vi "Host Main.vi"() -> ()   [LabVIEW 2014]
uses:
  rotate right.ctl
  rotate left.ctl
panel:
  in  "Rleft":T1
  in  "RRight":T2
  in  "Cancel Button":bool
  in  "Target IP Address":string="172.16.0.1"
  in  "Left Button":bool
  in  "Down Button":bool
  in  "Up Button":bool
  in  "Right Button":bool
  in  "Stop Button":bool
  # "Rover Demo (Host)"
  # "1. Confirm the IP address listed matches the WiFi IP address of the myRIO you are working with. Your myRIO has\ntwo different IP addresses, one for when it is connected through USB and another when it is broadcasting its own \nWiFi network.\n2. Open and Run the RT Main VI\n3. Run this VI\n4. Press all of the buttons and confirm they perform the appripriate movements."
  # "For help on troubleshooting this example as well as a brief description of how this example works \nvisit the help document under the My Computer section of the Project Viewer"
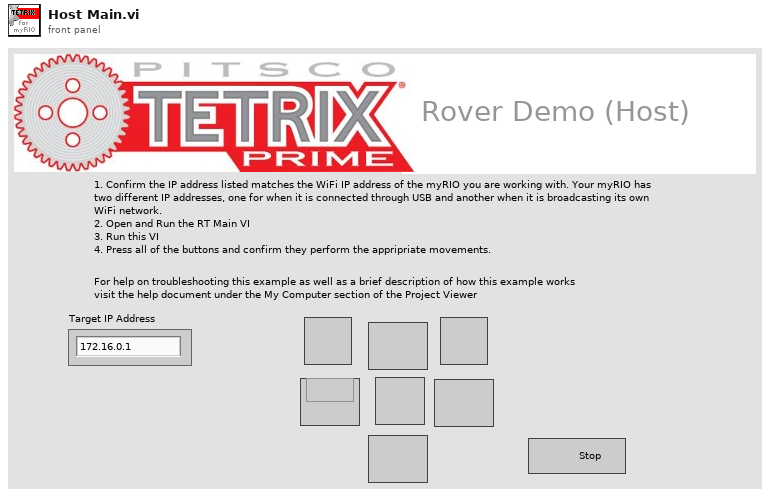
[diagram p1: front panel]
types:
  T1 = typedef "rotate left.ctl" = bool
  T2 = typedef "rotate right.ctl" = bool
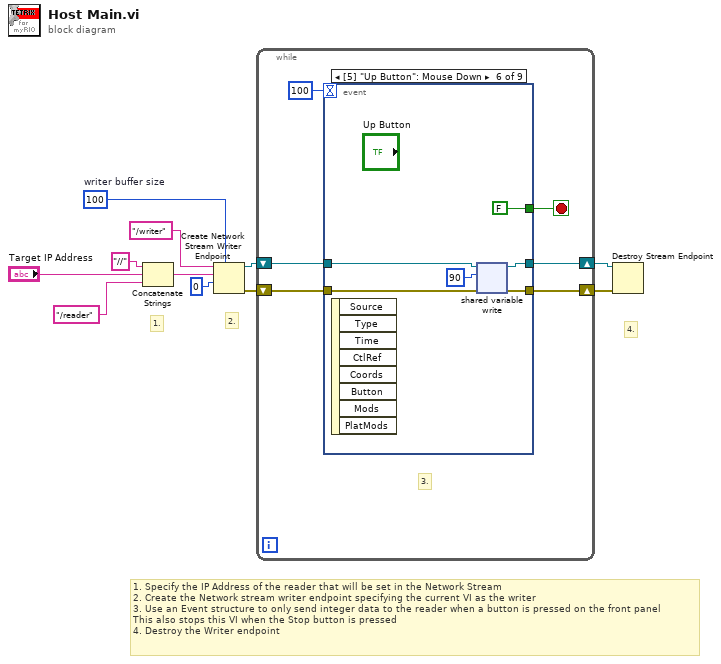
[diagram p0: block diagram]
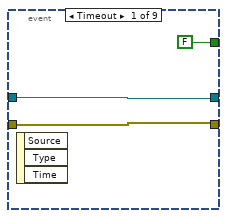
[diagram p2: hidden frame]
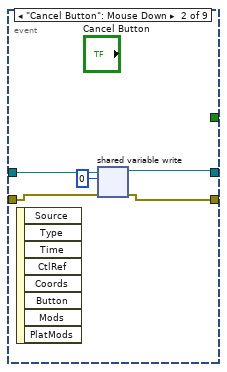
[diagram p3: hidden frame]
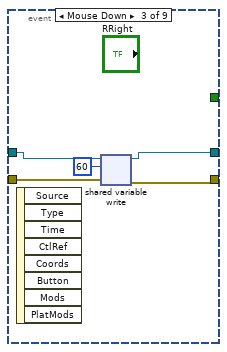
[diagram p4: hidden frame]
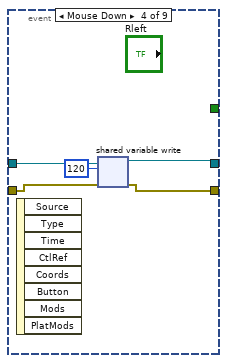
[diagram p5: hidden frame]
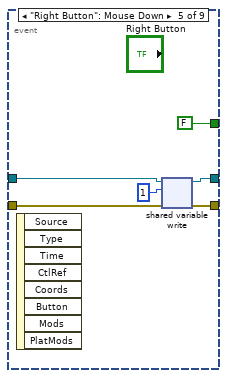
[diagram p6: hidden frame]
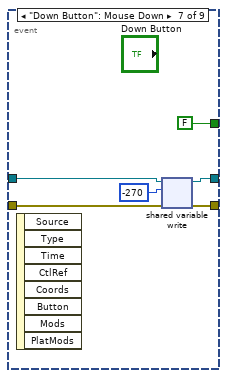
[diagram p7: hidden frame]
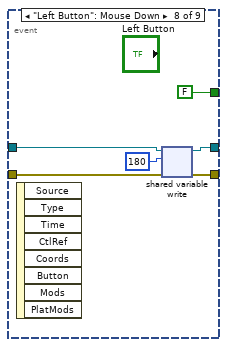
[diagram p8: hidden frame]
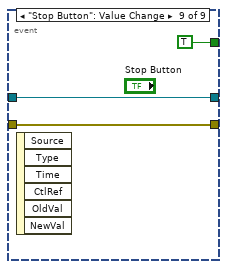
[diagram p9: hidden frame]
diagram:
  w11 = 100  # writer buffer size
  # "1. Specify the IP Address of the reader that will be set in the Network Stream\n2. Create the Network stream writer endpoint specifying the current VI as the writer\n3. Use an Event structure to only send integer data to the reader when a button is pressed on the front panel\nThis also stops this VI when the Stop button is pressed\n4. Destroy the Writer endpoint"
  # "4."
  # "2."
  # "1."
  n1 = Concatenate Strings("//", "Target IP Address", "/reader") -> (w10:string)
  n2 = Create Network Stream Writer Endpoint(7:w11, 9:0, 10:w10, 11:"/writer" ("reader name")) -> (0:w4:errorcluster, 3:w5:refnum<k21>)  [unwired: 3 in]
  n3 = while {
    shift-right: [w12] -> w1
    shift-left: w4 -> [w14]
    shift-right: [w13] -> w2
    shift-left: w5 -> [w15]
    stop <- w17 stop-if-true
    # "3."
    n4 = event shown="[5] \"Up Button\": Mouse Down" {
      selector: _ -> [_ _ _ _ _ _ _ _ _]
      dyn-events: _ -> [_ _ _ _ _ _ _ _ _]
      timeout: 100 -> [_ _ _ _ _ _ _ _ _]
      tunnel: [FALSE _ _ _ FALSE FALSE FALSE FALSE TRUE] -> w17
      tunnel: w15 -> [w19 w25 w30 w35 w40 w46 w52 w58 w61]
      tunnel: w14 -> [w18 w24 w28 w34 w39 w45 w51 w57 w60]
      tunnel: [w19 w23 w29 w33 w38 w44 w50 w56 w61] -> w13
      tunnel: [w18 w22 w27 w32 w37 w43 w49 w55 w60] -> w12
      event Timeout {
        n5 = event-data() -> ()  [unwired: 1 in, 3 out]
      }
      event "Cancel Button": Mouse Down {
        n6 = event-data() -> ()  [unwired: 1 in, 8 out]
        n7 = shared-variable-write(w25, w24, 0 ("data in")) -> (w23:refnum<k21>, w22:errorcluster)  [unwired: 1 in, 1 out]
      }
      event Mouse Down {
        n8 = event-data() -> ()  [unwired: 1 in, 8 out]
        n9 = shared-variable-write(w30, w28, 60 ("data in")) -> (w29:refnum<k21>, w27:errorcluster)  [unwired: 1 in, 1 out]
      }
      event Mouse Down {
        n10 = event-data() -> ()  [unwired: 1 in, 8 out]
        n11 = shared-variable-write(w35, w34, 120 ("data in")) -> (w33:refnum<k21>, w32:errorcluster)  [unwired: 1 in, 1 out]
      }
      event "Right Button": Mouse Down {
        n12 = event-data() -> ()  [unwired: 1 in, 8 out]
        n13 = shared-variable-write(w40, w39, 1 ("data in")) -> (w38:refnum<k21>, w37:errorcluster)  [unwired: 1 in, 1 out]
      }
      event "Up Button": Mouse Down {
        n14 = event-data() -> ()  [unwired: 1 in, 8 out]
        n15 = shared-variable-write(w46, w45, 90 ("data in")) -> (w44:refnum<k21>, w43:errorcluster)  [unwired: 1 in, 1 out]
      }
      event "Down Button": Mouse Down {
        n16 = event-data() -> ()  [unwired: 1 in, 8 out]
        n17 = shared-variable-write(w52, w51, -270 ("data in")) -> (w50:refnum<k21>, w49:errorcluster)  [unwired: 1 in, 1 out]
      }
      event "Left Button": Mouse Down {
        n18 = event-data() -> ()  [unwired: 1 in, 8 out]
        n19 = shared-variable-write(w58, w57, 180 ("data in")) -> (w56:refnum<k21>, w55:errorcluster)  [unwired: 1 in, 1 out]
      }
      event "Stop Button": Value Change {
        n20 = event-data() -> ()  [unwired: 1 in, 6 out]
      }
    }
  }
  n21 = Destroy Stream Endpoint(8:w1, 11:w2) -> ()  [unwired: 1 out]
